vi "Example1.vi"   [LabVIEW 2015]
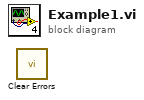
[diagram p0: block diagram]
diagram:
  n1 = call <vilib>:"Clear Errors.vi"() -> ()  [unwired: 6 in, 2 out]
